vi "Initialize.vi"(9 "Column":i32, 10 "Row":i32, 11 "Defenders in":refnum<class "Defenders.lvclass">) -> (3 "Defenders out":refnum<class "Defenders.lvclass">)   [LabVIEW 2015, in "Defenders.lvclass"]
uses:
  Defenders.lvclass
  Defenders.lvclass/Defenders.ctl
  Common/Common.lvlib
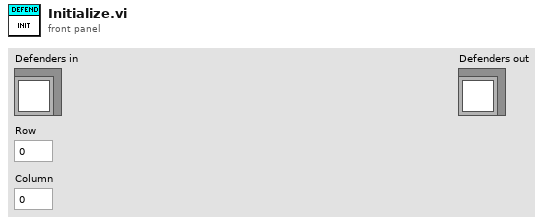
[diagram p1: front panel]
types:
  T1 = typedef "Common.lvlib/Map DVR.ctl" = refnum<data-value>
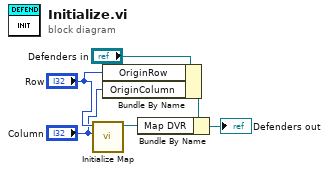
[diagram p0: block diagram]
diagram:
  n1 = call "Initialize Map.vi"("Column"="Column", "Row"="Row") -> ("Map DVR"=w4:T1)  [unwired: 9 in]
  n2 = Bundle By Name(cluster="Defenders in", "OriginRow"="Row", "OriginColumn"="Column") -> (w3:refnum<class "Defenders.lvclass">)
  n3 = Bundle By Name(cluster=w3, "Map DVR"=w4) -> (→"Defenders out":refnum<class "Defenders.lvclass">)
